vi "Move Z.vi"(8 "error in (no error)":errorcluster, 10 "Delta (um)":dbl, 11 "Stage Controller in":refnum<class "Stage Controller.lvclass">) -> (0 "error out":errorcluster, 3 "Stage Controller out":refnum<class "Stage Controller.lvclass">)   [LabVIEW 2018, in "Stage Controller.lvlib" / "Stage Controller.lvclass"]
uses:
  Stage Controller.lvclass
  Microscope/ti2lv/ti2lv.lvlib
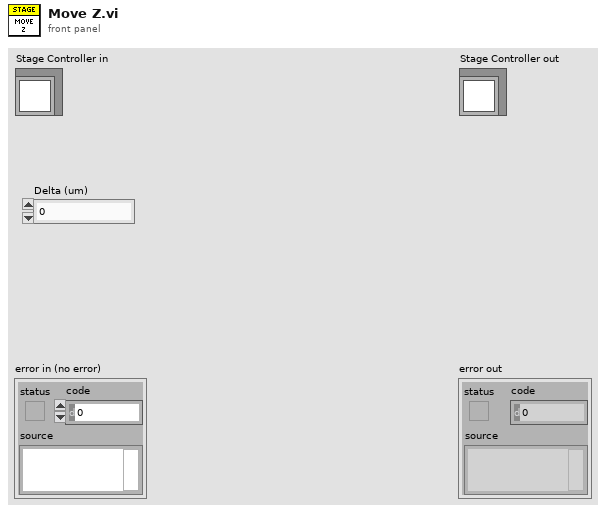
[diagram p1: front panel]
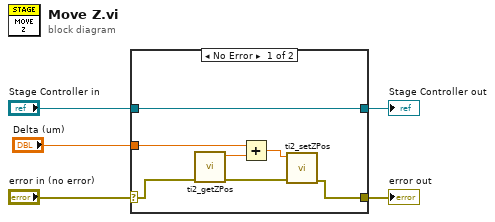
[diagram p0: block diagram]
diagram:
  n1 = case shown="No Error" "error in (no error)" {
    selector: "error in (no error)" -> [w11 w14]
    tunnel: [w9 w14] -> w4
    tunnel: [w12 w13] -> w2
    tunnel: "Stage Controller in" -> [w12 w13]
    tunnel: "Delta (um)" -> [w8 _]
    frame No Error {
      n2 = call "ti2_getZPos.vi"("error in (no error)"=w11) -> ("error out"=w10:errorcluster, "z Position (um)"=w7:dbl)  [unwired: 9 in]
      n3 = Add(x=w8, y=w7) -> (x+y=w6:dbl)
      n4 = call "ti2_setZPos.vi"("error in (no error)"=w10, "z Position (um)"=w6) -> ("error out"=w9:errorcluster)  [unwired: 9 in]
    }
    frame Error {
    }
  }
  "error out" <- w4
  "Stage Controller out" <- w2
